vi "niRFUtil CONV 1 Ohm Voltage to dBm (real scalar).vi"(7 "Real Scalar (V)":sgl format="%.2f") -> (8 "Real Scalar (dBm)":sgl format="%.2f")   [LabVIEW 2015, in "niRFUtil.lvlib"]
doc: "(c) Copyright 2006, National Instruments, Inc. This VI may not be duplicated, sold, or distributed without written consent from National Instruments."
uses:
  niRFUtil.lvlib
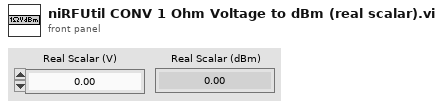
[diagram p1: front panel]
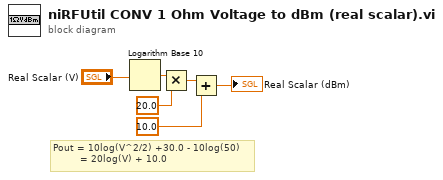
[diagram p0: block diagram]
diagram:
  # "Pout = 10log(V^2/2) +30.0 - 10log(50)\n         = 20log(V) + 10.0"
  n1 = Logarithm Base 10(1:"Real Scalar (V)") -> (0:w6:sgl)
  n2 = Multiply(x=w6, y=sgl 20.0) -> (x*y=w4:sgl)
  n3 = Add(x=w4, y=sgl 10.0) -> (x+y=→"Real Scalar (dBm)":sgl)
